vi "Save Graphic.vi"(6 "Loc string caption":string, 7 "FP Title":string, 8 "error in (no error)":errorcluster, 11 "Start path in":path) -> (0 "error out":errorcluster, 3 "Output":path)   [LabVIEW 2021]
doc: "<p>Select <strong>File<span class=\"U+187\">>></span>Save As<span class=\"U+187\">>></span>Template</strong> or <strong>File<span class=\"U+187\">>></span>Save As<span class=\"U+187\">>></span>Glyph</strong> from the <a href=\"nihelplauncher://docs/csh?context=lvcore_lvdialog_icon_editor\">Icon Editor</a> dialog box to display this dialog box. Depending on the <strong>File</strong> menu item you select, the title of this dialog box appears as either <strong>Save Icon Template</strong> or <strong>Save Glyph</strong>.</p>\n<p>Use this dialog box to save an <a href=\"nihelplauncher://docs/csh?context=lvcore_lvconcepts_using_icons\">icon</a> you <a href=\"nihelplauncher://docs/csh?context=lvcore_lvhowto_creating_vi_icon\">create</a> as a template or glyph for later use. You must save icon templates within the <span class=\"Monospace\">LabVIEW Data\\Icon Templates</span> directory. You must save glyphs within the <span class=\"Monospace\">LabVIEW Data\\Glyphs</span> directory. LabVIEW saves icon templates and glyphs you create in the <strong>Icon Editor</strong> dialog box as 256-color <span class=\"Monospace\">.png</span> files.</p>\n<p>This dialog box includes the following components:</p>"
uses:
  <vilib>/Utility/miscctls.llb/LVRowAndColumnTypeDef.ctl
  <vilib>/Utility/error.llb/Trim Whitespace One-Sided.vi
  <vilib>/Utility/Multibyte/NI_Multibyte Utilities.lvlib
panel:
  in  "Rename":string="Rename"
  in  "Name":string caption="Glyph name"
  in  "Tree":string(tree)="C:\\Documents and Settings\\grsandrt\\My Documents\\LabVIEW Data\\Icon Templates\\Library\\Frameworks\\New Folder\\New Folder\\New Folder\\New Folder\\New Folder\\New Folder\\New Folder\\New Folder\\New Folder 35"
  in  "Loc string":string[](array[string])=["Folder Structure"]
  in  "New folder":bool
  in  "Help":bool
  in  "Cancel":bool
  in  "Save":bool
  in  "New folder":string="New Folder"
  out "Final path":path
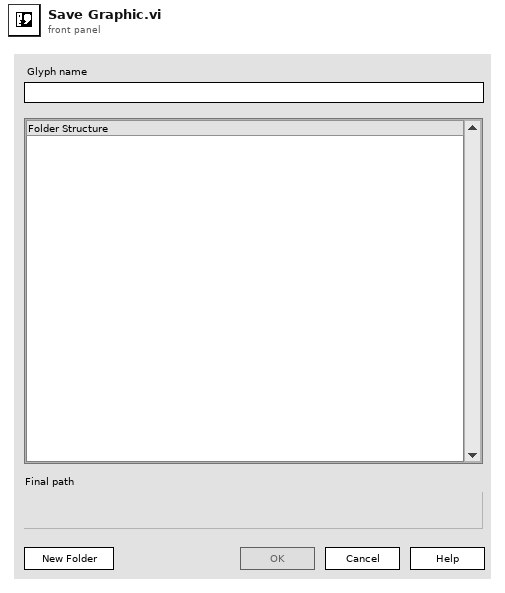
[diagram p1: front panel]
types:
  T1 = enum32{"Invalid", "Standard", "Closed", "Hidden", "Minimized", "Maximized"}
  T2 = typedef "LVRowAndColumnTypeDef.ctl" = cluster{"Row":i32, "Column":i32}
  T3 = typedef "LVPoint32TypeDef.ctl" = cluster{"Horizontal":i32, "Vertical":i32}
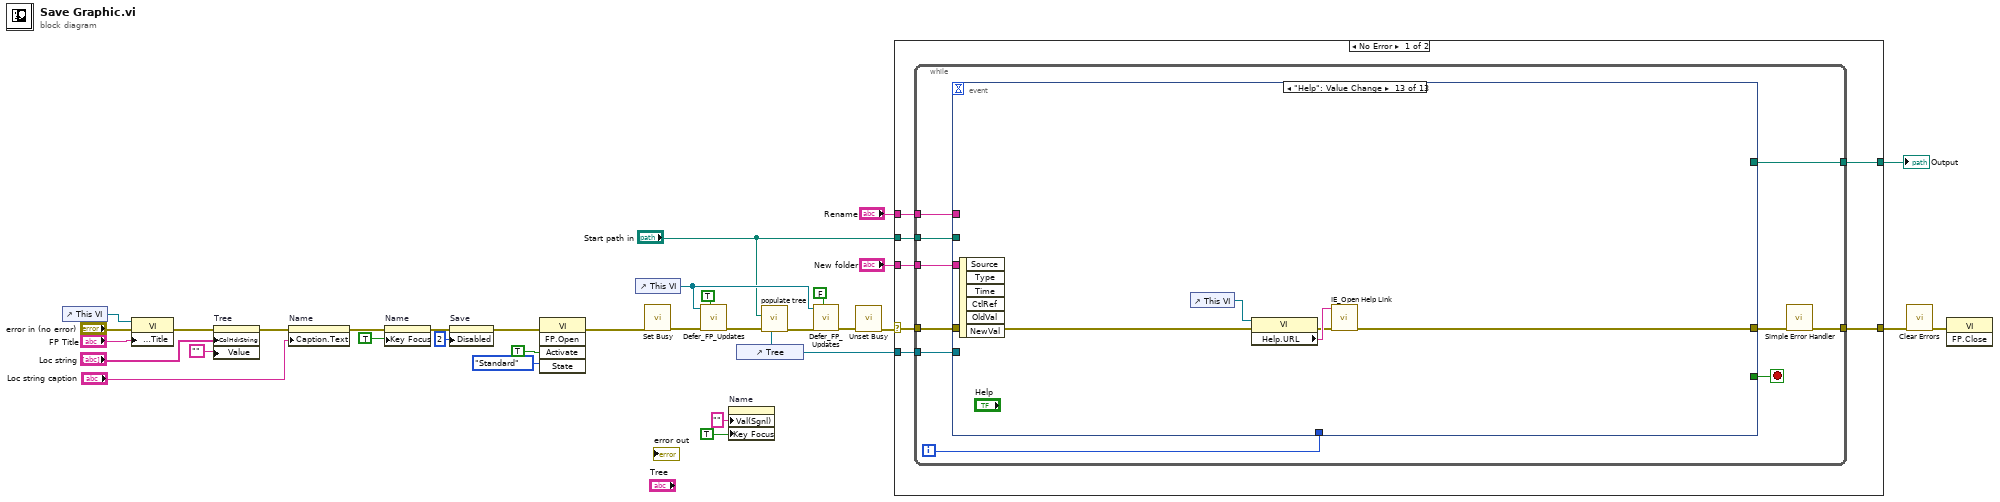
[diagram p0: block diagram]
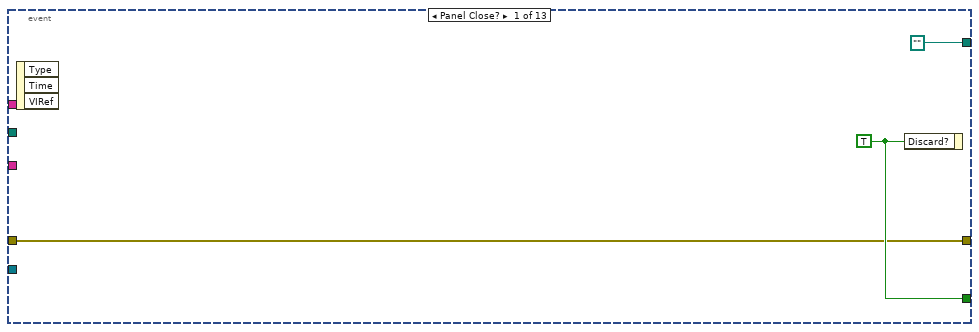
[diagram p2: hidden frame]
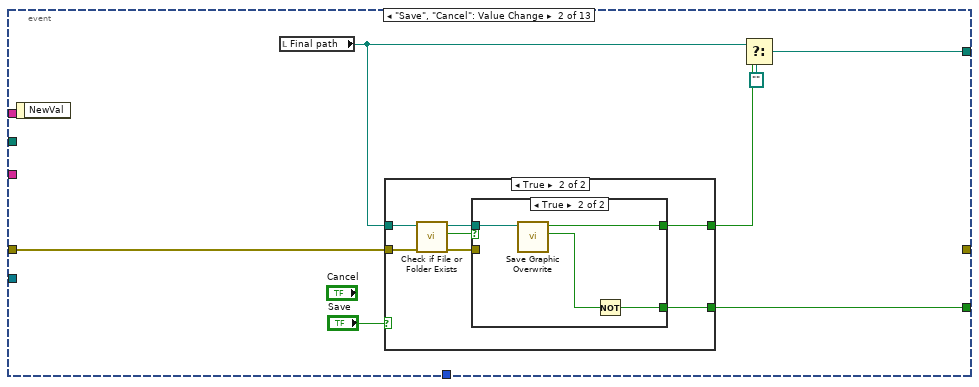
[diagram p3: hidden frame]
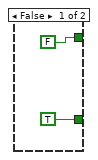
[diagram p4: hidden frame]
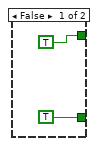
[diagram p5: hidden frame]
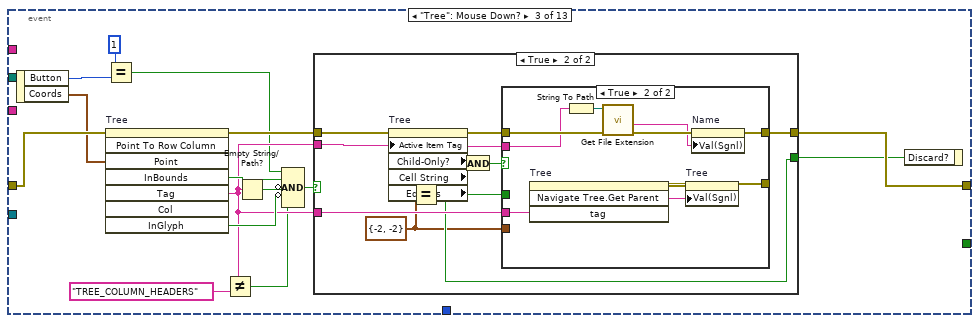
[diagram p6: hidden frame]
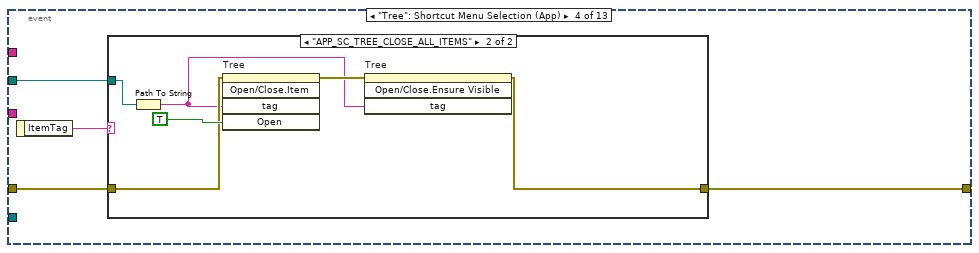
[diagram p9: hidden frame]
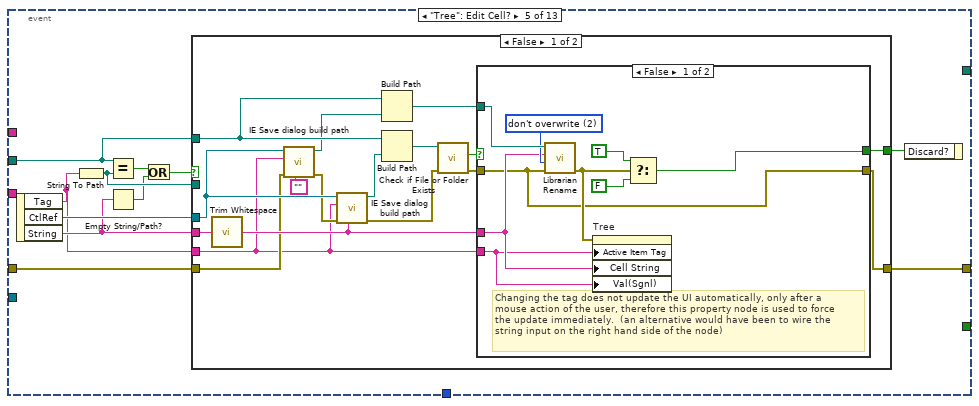
[diagram p11: hidden frame]
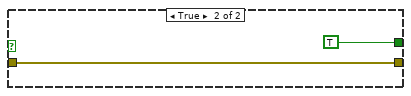
[diagram p12: hidden frame]
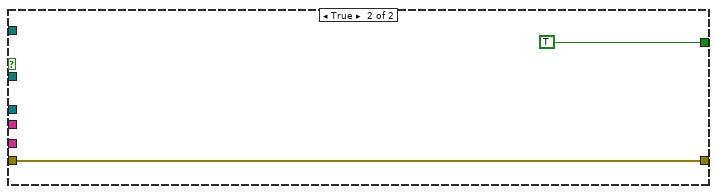
[diagram p13: hidden frame]
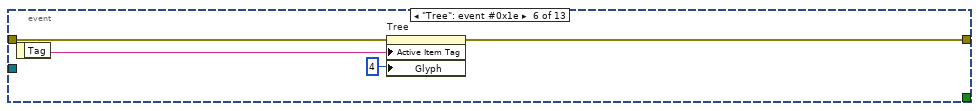
[diagram p14: hidden frame]
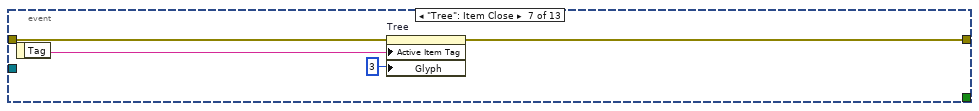
[diagram p15: hidden frame]
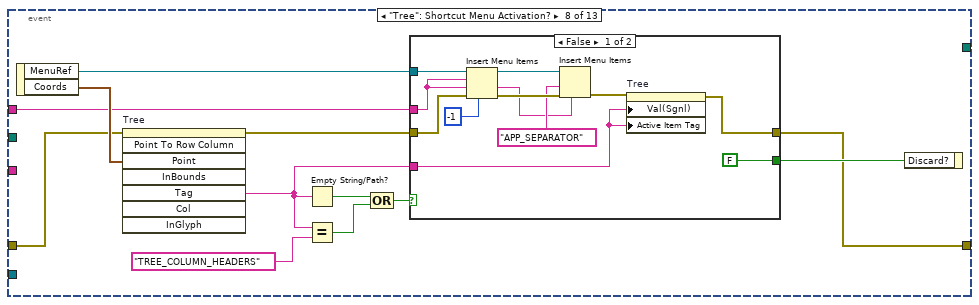
[diagram p16: hidden frame]
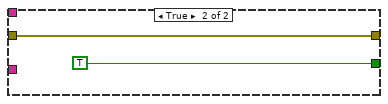
[diagram p17: hidden frame]
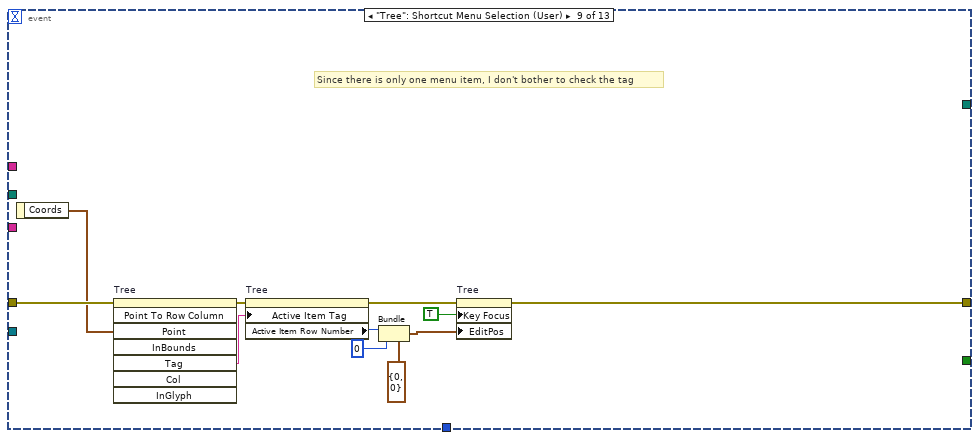
[diagram p18: hidden frame]
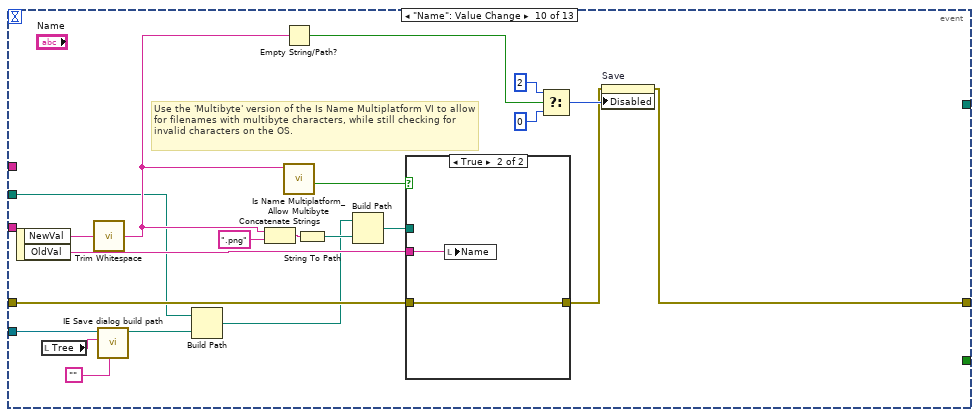
[diagram p19: hidden frame]
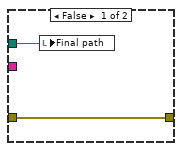
[diagram p20: hidden frame]
diagram:
  n1 = control-ref of="This VI"() -> (w25:refnum<vi>)
  n2 = property class="VI"(reference=w25, error in="error in (no error)", "Front Panel.Title"="FP Title") -> (error out=w26:errorcluster)  [unwired: 1 out]
  n3 = property on="Tree" class="Tree (strict)"(error in=w26, "ColHdrString"="Loc string", "Value"="") -> (error out=w3:errorcluster)  [unwired: 1 in, 1 out]
  n4 = property on="Name" class="Str"(error in=w3, "Caption.Text"="Loc string caption") -> (error out=w4:errorcluster)  [unwired: 1 in, 1 out]
  n5 = property on="Name" class="Str"(error in=w4, "Key Focus"=TRUE) -> (error out=w29:errorcluster)  [unwired: 1 in, 1 out]
  n6 = property on="Save" class="Bool"(error in=w29, "Disabled"=u8 2) -> (error out=w9:errorcluster)  [unwired: 1 in, 1 out]
  n7 = invoke class="VI" method="FP.Open"(error in=w9, "Activate"=TRUE ("Activate?"), "State"=T1."Standard") -> (error out=w13:errorcluster)  [unwired: 2 in, 4 out]
  n8 = control-ref of="This VI"() -> (w19:refnum<vi>)
  n9 = call <vilib>:"Set Busy.vi"("error in (no error)"=w13) -> ("error out"=w17:errorcluster)  [unwired: 3 in, 7 out]
  n10 = call "Defer_FP_Updates.vi"("Defer Panel Updates"=TRUE, "error in (no error)"=w17, "lv_icon.vi in"=w19) -> ("error out"=w21:errorcluster)  [unwired: 8 out]
  n11 = property on="Name" class="Str"("Val(Sgnl)"="" ("Glyph name"), "Key Focus"=TRUE) -> ()  [unwired: 2 in, 2 out]
  n12 = control-ref of="Tree"() -> (w10:refnum<vi>)
  n13 = call "populate tree.vi"("Tree Refnum"=w10, "error in (no error)"=w21, "Root"="Start path in") -> ("error out"=w20:errorcluster)  [unwired: 1 in, 7 out]
  n14 = call "Defer_FP_Updates.vi"("Defer Panel Updates"=FALSE, "error in (no error)"=w20, "lv_icon.vi in"=w19) -> ("error out"=w16:errorcluster)  [unwired: 8 out]
  n15 = call <vilib>:"Unset Busy.vi"("error in (no error)"=w16) -> ("error out"=w15:errorcluster)  [unwired: 1 in, 9 out]
  n16 = case shown="No Error" w15 {
    selector: w15 -> [w39 _]
    tunnel: "New folder" -> [w40 _]
    tunnel: "Start path in" -> [w38 _]
    tunnel: [w37 _] -> w14
    tunnel: w10 -> [w36 _]
    tunnel: [w35 _] -> w7
    tunnel: "Rename" -> [w34 _]
    frame No Error {
      n17 = while {
        tunnel: w40 -> [w46]
        tunnel: w38 -> [w48]
        tunnel: [w47] -> w37
        tunnel: w39 -> [w49]
        tunnel: w36 -> [w44]
        tunnel: [w42] -> w35
        tunnel: w34 -> [w41]
        i -> [w43]
        stop <- w50 stop-if-true
        n18 = event shown="[12] \"Help\": Value Change" {
          selector: _ -> [_ _ _ _ _ _ _ _ _ _ _ _ _]
          dyn-events: _ -> [_ _ _ _ _ _ _ _ _ _ _ _ _]
          timeout: _ -> [_ _ _ _ _ _ _ _ _ _ _ _ _]
          tunnel: [w53 w56 _ _ _ _ _ _ _ _ _ _ _] -> w50
          tunnel: [w52 _ w85 w114 w133 w167 w171 w178 w200 w228 w252 w265 w289] -> w45
          tunnel: w49 -> [w52 w58 w90 w115 w134 w168 w172 w182 w203 w220 w242 w263 w292]
          tunnel: w48 -> [_ _ _ w116 w130 _ _ _ _ w212 w240 w256 _]
          tunnel: [path "" w60 _ _ _ _ _ _ _ _ _ _ _] -> w47
          tunnel: w46 -> [_ _ _ _ _ _ _ _ _ _ _ w275 _]
          tunnel: w44 -> [_ _ _ _ _ _ _ _ _ w217 _ w264 _]
          tunnel: w43 -> [_ _ _ _ _ _ _ _ _ _ _ w260 _]
          tunnel: w41 -> [_ _ _ _ _ _ _ w180 _ _ _ _ _]
          event Panel Close? {
            w53 = TRUE ("Discard?")
            n19 = event-data() -> ()  [unwired: 4 out]
            n20 = event-data("Discard?"=w53) -> ()  [unwired: 1 in, 1 out]
          }
          event "Save", "Cancel": Value Change {
            n21 = event-data() -> ()  [unwired: 2 out]
            n22 = local read "Final path"() -> (w55:path)
            n23 = case shown="True" "Save" {
              tunnel: w58 -> [_ w69]
              tunnel: [TRUE w66] -> w56
              tunnel: w55 -> [_ w65]
              tunnel: [FALSE w64] -> w54
              frame False {
              }
              frame True {
                n24 = call <vilib>:"Check if File or Folder Exists.vi"("error in (no error)"=w69, "path"=w65) -> ("error out"=w67:errorcluster, "file or folder exists?"=w68:bool, "dup path"=w63:path)  [unwired: 7 in]
                n25 = case shown="True" w68 {
                  tunnel: w67 -> [_ _]
                  tunnel: [TRUE w73] -> w66
                  tunnel: [TRUE w75] -> w64
                  tunnel: w63 -> [_ w72]
                  frame False {
                  }
                  frame True {
                    n26 = call "Save Graphic Overwrite.vi"("Path"=w72) -> ("Cancel"=w74:bool, "OK"=w75:bool)  [unwired: 9 in]
                    n27 = Not(x=w74) -> (.not. x?=w73:bool)
                  }
                }
              }
            }
            n28 = Select(t=w55, s=w54, f=path "") -> (s? t:f=w60:path)
          }
          event "Tree": Mouse Down? {
            n29 = event-data() -> ("Button"=w78:u16, "Coords"=w89:T3)  [unwired: 1 out]
            n30 = Equal?(x=u16 1, y=w78) -> (x = y?=w77:bool)
            n31 = invoke on="Tree" class="Tree (strict)" method="Point To Row Column"(error in=w90, "Point"=w89) -> (error out=w88:errorcluster, "InBounds"=w84:bool, "Tag"=w81:string, "InGlyph"=w83:bool)  [unwired: 6 in, 4 out]
            n32 = Not Equal?(x=w81, y="TREE_COLUMN_HEADERS") -> (x != y?=w79:bool)
            n33 = Empty String/Path?(string/path=w81) -> (empty?=w87:bool)
            n34 = Compound Arithmetic op=AND(w77, w84, invert w87, invert w83, w79) -> (w86:bool)
            n35 = case shown="True" w86 {
              tunnel: w88 -> [w91 w102]
              tunnel: w81 -> [_ w97]
              tunnel: [w91 w98] -> w85
              tunnel: w81 -> [_ w101]
              tunnel: [_ w94] -> w82
              frame False {
              }
              frame True {
                w92 = T2 {"Row"=-2, "Column"=-2} ("y")
                n36 = property on="Tree" class="Tree (strict)"(error in=w102, "Active Item Tag"=w101) -> (error out=w99:errorcluster, "Child-Only?"=w94:bool, "Cell String"=w100:string, "EditPos"=w96:T2)  [unwired: 1 in, 1 out]
                n37 = Equal?(x=w96, y=w92) -> (x = y?=w93:bool)
                n38 = And(x=w94, y=w93) -> (x .and. y?=w95:bool)
                n39 = case shown="True" w95 {
                  tunnel: w100 -> [_ w109]
                  tunnel: w99 -> [w103 w112]
                  tunnel: [w103 w113] -> w98
                  tunnel: w97 -> [_ w105]
                  tunnel: [_ w104] -> _
                  tunnel: w93 -> [_ _]
                  tunnel: w92 -> [_ _]
                  frame False {
                  }
                  frame True {
                    n40 = invoke on="Tree" class="Tree (strict)" method="Navigate Tree.Get Parent"("tag"=w105) -> (error out=w106:errorcluster, "Navigate Tree:Get Parent"=w107:string)  [unwired: 3 in, 2 out]
                    n41 = String To Path(string=w109) -> (path=w108:path)
                    n42 = call <vilib>:"Get File Extension.vi"("error in (no error)"=w112, "file"=w108) -> ("error out"=w111:errorcluster, "filename without extension"=w110:string)  [unwired: 8 out]
                    n43 = property on="Tree" class="Tree (strict)"(error in=w106, "Val(Sgnl)"=w107) -> (error out=w104:errorcluster)  [unwired: 1 in, 1 out]
                    n44 = property on="Name" class="Str"(error in=w111, "Val(Sgnl)"=w110) -> (error out=w113:errorcluster)  [unwired: 1 in, 1 out]
                  }
                }
              }
            }
            n45 = event-data("Discard?"=w82) -> ()  [unwired: 1 in, 1 out]
          }
          event "Tree": Shortcut Menu Selection (App) {
            n46 = event-data() -> ("ItemTag"=w117:string)  [unwired: 1 out]
            n47 = case shown="\"APP_SC_TREE_CLOSE_ALL_ITEMS\"" w117 {
              tunnel: w116 -> [_ w124]
              tunnel: w115 -> [w118 w122]
              tunnel: [w118 w119] -> w114
              frame "False", Default {
              }
              frame "APP_SC_TREE_CLOSE_ALL_ITEMS" {
                n48 = Path To String(path=w124) -> (string=w120:string)
                n49 = invoke on="Tree" class="Tree (strict)" method="Open/Close.Item"(error in=w122, "tag"=w120, "Open"=TRUE ("Open?")) -> (error out=w121:errorcluster)  [unwired: 2 in, 4 out]
                n50 = invoke on="Tree" class="Tree (strict)" method="Open/Close.Ensure Visible"(error in=w121, "tag"=w120) -> (error out=w119:errorcluster)  [unwired: 2 in, 3 out]
              }
            }
          }
          event "Tree": Edit Cell? {
            n51 = event-data() -> ("Tag"=w125:string, "CtlRef"=w135:refnum<vi>, "String"=w129:string)  [unwired: 1 out]
            n52 = String To Path(string=w125) -> (path=w131:path)
            n53 = Equal?(x=w130, y=w131) -> (x = y?=w128:bool)
            n54 = Empty String/Path?(string/path=w129) -> (empty?=w127:bool)
            n55 = Or(x=w128, y=w127) -> (x .or. y?=w126:bool)
            n56 = case shown="False" w126 {
              tunnel: w129 -> [w152 _]
              tunnel: w130 -> [w139 _]
              tunnel: w135 -> [w144 _]
              tunnel: w134 -> [w143 w164]
              tunnel: [w146 w164] -> w133
              tunnel: [w145 TRUE] -> w132
              tunnel: w131 -> [_ _]
              tunnel: w125 -> [w136 _]
              frame False {
                n57 = call <vilib>:"Trim Whitespace.vi"("string"=w152) -> ("trimmed string"=w147:string)  [unwired: 1 in]
                n58 = call "IE Save dialog build path.vi"("New String"="", "error in (no error)"=w143, "Start tag"=w136, "Tree Refnum"=w144) -> ("error out"=w142:errorcluster, "New path"=w138:path)  [unwired: 6 out]
                n59 = call "IE Save dialog build path.vi"("New String"=w147, "error in (no error)"=w142, "Start tag"=w136, "Tree Refnum"=w144) -> ("error out"=w150:errorcluster, "New path"=w151:path)  [unwired: 6 out]
                n60 = Build Path(base path=w139, name or relative path=w138) -> (appended path=w137:path)
                n61 = Build Path(base path=w139, name or relative path=w151) -> (appended path=w140:path)
                n62 = call <vilib>:"Check if File or Folder Exists.vi"("error in (no error)"=w150, "path"=w140) -> ("error out"=w148:errorcluster, "file or folder exists?"=w149:bool)  [unwired: 8 out]
                n63 = case shown="False" w149 {
                  tunnel: w148 -> [w154 w163]
                  tunnel: w147 -> [w155 _]
                  tunnel: [w154 w163] -> w146
                  tunnel: [w158 TRUE] -> w145
                  tunnel: w137 -> [w161 _]
                  tunnel: w136 -> [w153 _]
                  frame False {
                    w160 = u16 2 items=["overwrite", "ask first", "don't overwrite"] ("overwrite")
                    # "Changing the tag does not update the UI automatically, only after a\nmouse action of the user, therefore this property node is used to force\nthe update immediately.  (an alternative would have been to wire the\nstring input on the right hand side of the node)"
                    n64 = call <vilib>:"Librarian Rename.vi"("error in (no error)"=w154, "overwrite"=w160, "new name"=w155, "path"=w161) -> ("error out"=w156:errorcluster)  [unwired: 7 out]
                    n65 = property on="Tree" class="Tree (strict)"(error in=w156, "Active Item Tag"=w153, "Cell String"=w155, "Val(Sgnl)"=w153) -> ()  [unwired: 1 in, 2 out]
                    n66 = Select(t=TRUE, s=w156, f=FALSE) -> (s? t:f=w158:bool)
                  }
                  frame True {
                  }
                }
              }
              frame True {
              }
            }
            n67 = event-data("Discard?"=w132) -> ()  [unwired: 1 in, 1 out]
          }
          event "Tree": event #0x1e {
            n68 = event-data() -> ("Tag"=w166:string)  [unwired: 1 out]
            n69 = property on="Tree" class="Tree (strict)"(error in=w168, "Active Item Tag"=w166, "Glyph"=4 ("Active Item:Symbol Index")) -> (error out=w167:errorcluster)  [unwired: 1 in, 1 out]
          }
          event "Tree": Item Close {
            n70 = event-data() -> ("Tag"=w170:string)  [unwired: 1 out]
            n71 = property on="Tree" class="Tree (strict)"(error in=w172, "Active Item Tag"=w170, "Glyph"=3 ("Active Item:Symbol Index")) -> (error out=w171:errorcluster)  [unwired: 1 in, 1 out]
          }
          event "Tree": Shortcut Menu Activation? {
            n72 = event-data() -> ("MenuRef"=w185:refnum<k9>, "Coords"=w184:T3)  [unwired: 1 out]
            n73 = invoke on="Tree" class="Tree (strict)" method="Point To Row Column"(error in=w182, "Point"=w184) -> (error out=w181:errorcluster, "Tag"=w176:string)  [unwired: 6 in, 6 out]
            n74 = Empty String/Path?(string/path=w176) -> (empty?=w183:bool)
            n75 = Equal?(x=w176, y="TREE_COLUMN_HEADERS") -> (x = y?=w175:bool)
            n76 = Compound Arithmetic op=OR(w183, w175) -> (w177:bool)
            n77 = case shown="False" w177 {
              tunnel: w185 -> [w197 _]
              tunnel: w181 -> [w196 w198]
              tunnel: w176 -> [w186 _]
              tunnel: w180 -> [w195 _]
              tunnel: [FALSE TRUE] -> w179
              tunnel: [w187 w198] -> w178
              frame False {
                n78 = Insert Menu Items(4:-1, 6:w196, 7:w195, 8:w195, 9:w197) -> (0:w191:errorcluster, 1:w189:string, 3:w192:refnum<k9>)  [unwired: 1 in]
                n79 = Insert Menu Items(4:w189, 6:w191, 7:"APP_SEPARATOR", 9:w192) -> (0:w188:errorcluster)  [unwired: 2 in, 2 out]
                n80 = property on="Tree" class="Tree (strict)"(error in=w188, "Val(Sgnl)"=w186, "Active Item Tag"=w186) -> (error out=w187:errorcluster)  [unwired: 1 in, 1 out]
              }
              frame True {
              }
            }
            n81 = event-data("Discard?"=w179) -> ()  [unwired: 1 in, 1 out]
          }
          event "Tree": Shortcut Menu Selection (User) {
            # "Since there is only one menu item, I don't bother to check the tag"
            n82 = event-data() -> ("Coords"=w202:T3)  [unwired: 1 out]
            n83 = invoke on="Tree" class="Tree (strict)" method="Point To Row Column"(error in=w203, "Point"=w202) -> (error out=w204:errorcluster, "Tag"=w201:string)  [unwired: 6 in, 6 out]
            n84 = property on="Tree" class="Tree (strict)"(error in=w204, "Active Item Tag"=w201) -> (error out=w206:errorcluster, "Active Item Row Number"=w208:i32)  [unwired: 1 in, 1 out]
            n85 = Bundle(cluster=T2 {"Row"=0, "Column"=0} ("Edit Position"), "Row"=w208, "Column"=0) -> (w205:T2)
            n86 = property on="Tree" class="Tree (strict)"(error in=w206, "Key Focus"=TRUE, "EditPos"=w205) -> (error out=w200:errorcluster)  [unwired: 1 in, 1 out]
          }
          event "Name": Value Change {
            # "Use the 'Multibyte' version of the Is Name Multiplatform VI to allow for filenames with multibyte characters, while still checking for invalid characters on the OS."
            n87 = event-data() -> ("NewVal"=w226:string, "OldVal"=w231:string)  [unwired: 1 out]
            n88 = local read "Tree"() -> (w215:string)
            n89 = call <vilib>:"Trim Whitespace.vi"("string"=w226) -> ("trimmed string"=w224:string)  [unwired: 1 in]
            n90 = call "IE Save dialog build path.vi"("New String"="", "Start tag"=w215, "Tree Refnum"=w217) -> ("New path"=w213:path)  [unwired: 1 in, 7 out]
            n91 = Build Path(base path=w212, name or relative path=w213) -> (appended path=w211:path)
            n92 = Concatenate Strings(w224, ".png" ("string")) -> (w227:string)
            n93 = Empty String/Path?(string/path=w224) -> (empty?=w218:bool)
            n94 = call <vilib>:"Is Name Multiplatform_Allow Multibyte.vi"("filename"=w224) -> ("name had problem"=w229:bool)  [unwired: 7 in, 3 out]
            n95 = String To Path(string=w227) -> (path=w225:path)
            n96 = Build Path(base path=w211, name or relative path=w225) -> (appended path=w230:path)
            n97 = case shown="True" w229 {
              tunnel: w231 -> [_ w235]
              tunnel: w230 -> [w233 _]
              tunnel: w220 -> [w232 w234]
              tunnel: [w232 w234] -> w219
              frame False {
                n98 = local write "Final path"(w233) -> ()
              }
              frame True {
                n99 = local write "Name"(w235) -> ()
              }
            }
            n100 = Select(t=u8 2 ("Disabled"), s=w218, f=u8 0 ("Disabled")) -> (s? t:f=w221:u8)
            n101 = property on="Save" class="Bool"(error in=w219, "Disabled"=w221) -> (error out=w228:errorcluster)  [unwired: 1 in, 1 out]
          }
          event "Tree": Value Change {
            n102 = event-data() -> ("CtlRef"=w243:refnum<vi>, "NewVal"=w237:string)  [unwired: 1 out]
            n103 = call "IE Save dialog build path.vi"("New String"="", "error in (no error)"=w242, "Start tag"=w237, "Tree Refnum"=w243) -> ("error out"=w236:errorcluster, "New path"=w239:path)  [unwired: 6 out]
            n104 = local read "Name"() -> (w247:string)
            n105 = Build Path(base path=w240, name or relative path=w239) -> (appended path=w238:path)
            n106 = Concatenate Strings(w247, ".png" ("string")) -> (w251:string)
            n107 = Build Path(base path=w238, name or relative path=w251) -> (appended path=→"Final path":path)
            n108 = Empty String/Path?(string/path=w247) -> (empty?=w244:bool)
            n109 = Select(t=u8 2 ("Disabled"), s=w244, f=u8 0 ("Disabled")) -> (s? t:f=w246:u8)
            n110 = property on="Save" class="Bool"(error in=w236, "Disabled"=w246) -> (error out=w252:errorcluster)  [unwired: 1 in, 1 out]
          }
          event "New folder": Value Change {
            # "We have to make sure that\nthe tag is unique."
            # "Get next available unused folder name"
            n111 = event-data() -> ()  [unwired: 2 out]
            n112 = local read "Tree"() -> (w254:string)
            n113 = call "IE Save dialog build path.vi"("New String"="", "error in (no error)"=w263, "Start tag"=w254, "Tree Refnum"=w264) -> ("error out"=w262:errorcluster, "New path"=w255:path)  [unwired: 6 out]
            n114 = Build Path(base path=w256, name or relative path=w255) -> (appended path=w257:path)
            n115 = while {
              tunnel: w257 -> [w284]
              shift-right: [w281] -> w273
              shift-left: w262 -> [w282]
              tunnel: [w279] -> w274
              tunnel: w275 -> [w278]
              tunnel: [w276] -> w271
              i -> [w277]
              stop <- w280 continue-if-true
              n116 = case shown="0" w277 {
                selector: w277 -> [_ w288]
                tunnel: w278 -> [w285 w287]
                tunnel: [w285 w286] -> w276
                frame 0 {
                }
                frame 1, Default {
                  n117 = Format Into String(w287, w288) -> (resulting string=w286:string)  [unwired: 3 in, 1 out]
                }
              }
              n118 = Build Path(base path=w284, name or relative path=w276) -> (appended path=w283:path)
              n119 = call <vilib>:"Check if File or Folder Exists.vi"("error in (no error)"=w282, "path"=w283) -> ("error out"=w281:errorcluster, "file or folder exists?"=w280:bool, "dup path"=w279:path)  [unwired: 7 out]
            }
            n120 = call <vilib>:"Create Directory Recursive.vi"("error in (no error)"=w273, "directory"=w274) -> ("error out"=w253:errorcluster, "directory copy"=w261:path)  [unwired: 1 in, 3 out]
            n121 = Format Into String(w261, w260) -> (resulting string=w259:string)  [unwired: 3 in, 1 out]
            n122 = invoke on="Tree" class="Tree (strict)" method="Edit Tree Items.Add Item"(error in=w253, "Parent Tag"=w254, "Child Position"=0, "Left Cell"=w271, "Child Tag"=w259, "Child Only?"=FALSE) -> (error out=w269:errorcluster, "Edit Tree Items:Add Item"=w266:string)  [unwired: 3 in, 7 out]
            n123 = property on="Tree" class="Tree (strict)"(error in=w269, "Active Item Tag"=w266, "Val(Sgnl)"=w266, "Glyph"=3 ("Active Item:Symbol Index")) -> (error out=w267:errorcluster)  [unwired: 1 in, 1 out]
            n124 = invoke on="Tree" class="Tree (strict)" method="Open/Close.Ensure Visible"(error in=w267, "tag"=w266) -> (error out=w265:errorcluster)  [unwired: 2 in, 3 out]
          }
          event "Help": Value Change {
            n125 = event-data() -> ()  [unwired: 7 out]
            n126 = control-ref of="This VI"() -> (w293:refnum<vi>)
            n127 = property class="VI"(reference=w293, error in=w292) -> (error out=w290:errorcluster, "Help.URL"=w291:string)  [unwired: 1 out]
            n128 = call "IE_Open Help Link.vi"("error in (no error)"=w290, "Help.URL"=w291) -> ("error out"=w289:errorcluster)  [unwired: 9 in]
          }
        }
        n129 = call <vilib>:"Simple Error Handler.vi"("error in (no error)"=w45) -> ("error out"=w42:errorcluster)  [unwired: 1 in, 7 out]
      }
    }
    frame Error {
    }
  }
  "Output" <- w14
  n130 = call <vilib>:"Clear Errors.vi"("error in (no error)"=w7) -> ("error out"=w6:errorcluster)  [unwired: 5 in, 1 out]
  n131 = invoke class="VI" method="FP.Close"(error in=w6) -> ()  [unwired: 2 in, 3 out]
